vi "SetPos.vi"(1 "A":dbl format="%.4f", 2 "Z":dbl format="%.4f", 3 "Y":dbl format="%.4f", 4 "X":dbl format="%.4f") -> (0 "Command executed":bool)   [LabVIEW 2015, in "DelayLineLS4.lvclass"]
uses:
  Classes/Delay Line/DelayLineLS4/DelayLineLS4.lvclass
  DLL/LStep4.dll
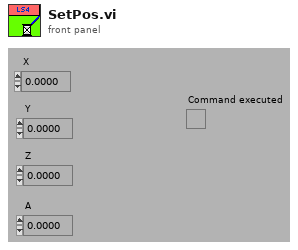
[diagram p1: front panel]
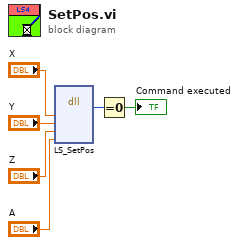
[diagram p0: block diagram]
diagram:
  n1 = dll-call lib="G:/SD/TRANCON/DLL/LStep4.dll" fn="LS_SetPos"("X"="X", "Y"="Y", "Z"="Z", "A"="A") -> ("type de retour"=w2:i32)  [unwired: 7 in, 2 out]
  n2 = Equal To 0?(x=w2) -> (x = 0?=→"Command executed":bool)
